vi "Unflatten (offset).vi"(8 "error in (no error)":errorcluster, 9 "offset (0)":i32, 10 "JSON stream":string, 11 "JSON Scalar in":refnum<class "JSON Scalar.lvclass">) -> (0 "error out":errorcluster, 1 "offset":i32, 3 "JSON Scalar out":refnum<class "JSON Scalar.lvclass">, 4 "Empty?":bool)   [LabVIEW 2020, in "Library Commun.lvlib" / "JSON Scalar.lvclass"]
uses:
  JSON Scalar.lvclass
  <vilib>/Utility/error.llb/whitespace.ctl
  JSON Scalar.lvclass/JSON Scalar.ctl
  support/JSON support.lvlib
  JSON Value/JSON Value.lvclass
panel:
  out "trimmed string":string
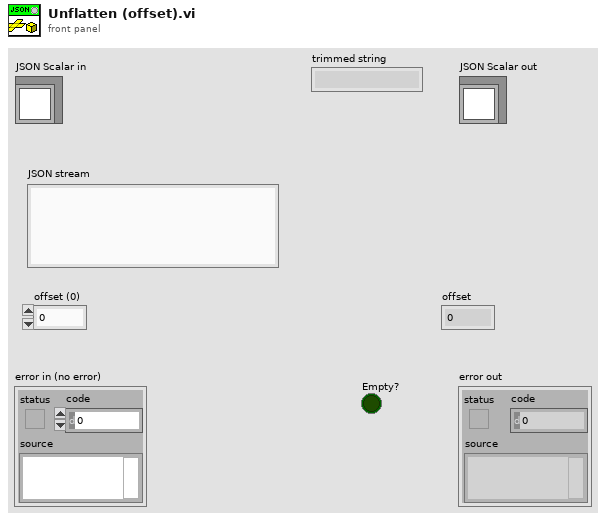
[diagram p1: front panel]
types:
  T1 = typedef "whitespace.ctl" = u16
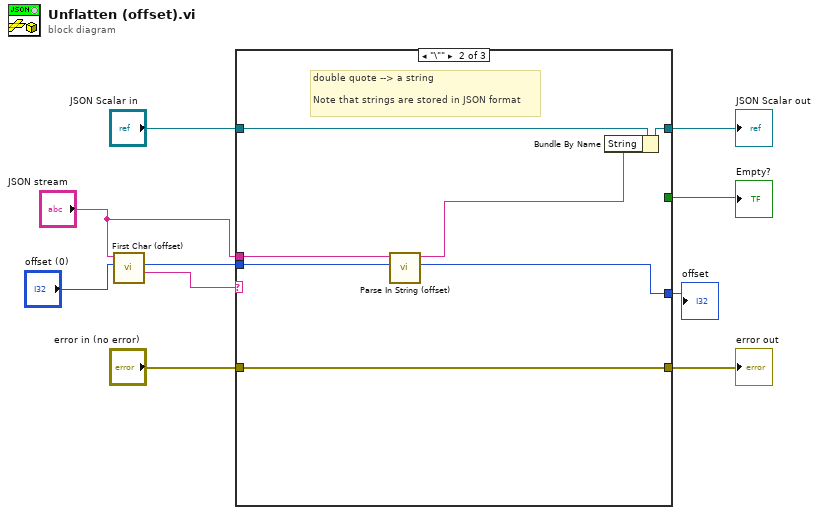
[diagram p0: block diagram]
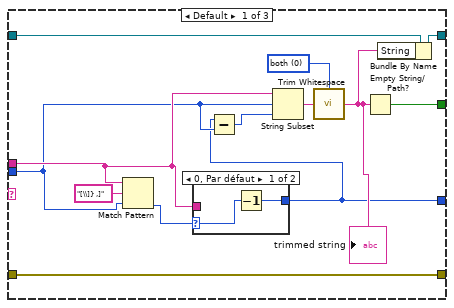
[diagram p2: hidden frame]
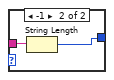
[diagram p3: hidden frame]
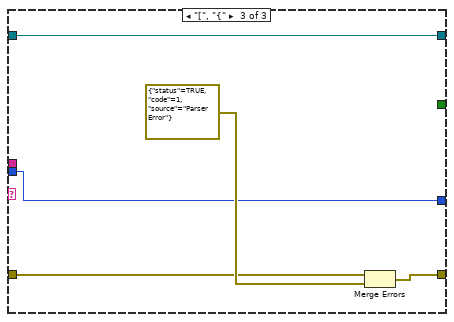
[diagram p4: hidden frame]
diagram:
  n1 = call "First Char (offset).vi"("offset (0)"="offset (0)", "String in"="JSON stream") -> ("First Char"=w4:string, "Offset"=w3:i32)  [unwired: 8 in]
  n2 = case shown="\"\\\"\"" w4 {
    tunnel: "error in (no error)" -> [w23 w30 w36]
    tunnel: [w23 w30 w39] -> w9
    tunnel: "JSON stream" -> [w15 w31 _]
    tunnel: [w20 w33 w38] -> w8
    tunnel: "JSON Scalar in" -> [w21 w34 w38]
    tunnel: [w17 _ _] -> w6
    tunnel: w3 -> [w13 w29 w35]
    tunnel: [w11 w28 w35] -> w2
    frame Default {
      w19 = T1 0 items=["both", "start of string", "end of string"] ("location (both)")
      n3 = Match Pattern(string=w15, regular expression="[\\]} ,]", offset (0)=w13) -> (offset past match=w16:i32)  [unwired: 3 out]
      n4 = case shown="0, Par défaut" w16 {
        selector: w16 -> [w25 _]
        tunnel: [w24 w26] -> w11
        tunnel: w15 -> [_ w27]
        frame 0, Default {
          n5 = Decrement(x=w25) -> (x-1=w24:i32)
        }
        frame -1 {
          n6 = String Length(string=w27) -> (length=w26:i32)
        }
      }
      n7 = Subtract(x=w11, y=w13) -> (x-y=w12:i32)
      n8 = String Subset(string=w15, offset (0)=w13, length (rest)=w12) -> (substring=w14:string)
      n9 = call <vilib>:"Trim Whitespace.vi"("string"=w14, "location (both)"=w19) -> ("trimmed string"=w18:string)
      "trimmed string" <- w18
      n10 = Empty String/Path?(string/path=w18) -> (empty?=w17:bool)
      n11 = Bundle By Name(cluster=w21, "String"=w18) -> (w20:refnum<class "JSON Scalar.lvclass">)
    }
    frame "\"" {
      # "double quote --> a string\n\nNote that strings are stored in JSON format"
      n12 = call "Parse In String (offset).vi"("offset"=w29, "JSON (quote at offset)"=w31) -> ("offset"=w28:i32, "String (incl quotes)"=w32:string)  [unwired: 8 in]
      n13 = Bundle By Name(cluster=w34, "String"=w32) -> (w33:refnum<class "JSON Scalar.lvclass">)
    }
    frame "[", "{" {
      n14 = Merge Errors(w36, errorcluster {"status"=TRUE, "code"=1, "source"="Parser Error"} ("error in")) -> (w39:errorcluster)
    }
  }
  "error out" <- w9
  "JSON Scalar out" <- w8
  "Empty?" <- w6
  "offset" <- w2
